vi "read header.vi"(6 "max bytes per line":i32=2048, 7 "max lines":i32=1024, 8 "error in (no error)":errorcluster, 11 "TCP Network Connection in":refnum<k5>) -> (0 "error out":errorcluster, 2 "header content":string, 3 "TCP Network Connection out":refnum<k5>)   [LabVIEW 2019, in "WebSocket Server Toolkit.lvlib"]
uses:
  WebSocket Server Toolkit.lvlib
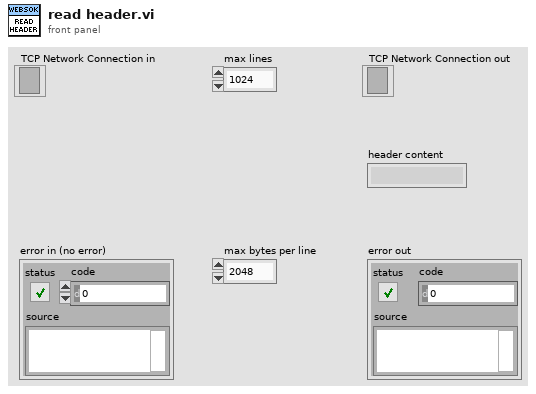
[diagram p1: front panel]
types:
  T1 = enum16{"Standard", "Buffered", "CRLF", "Immediate"}
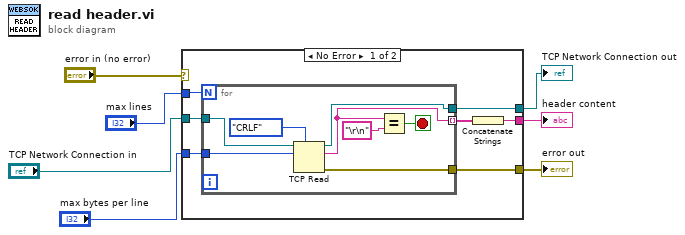
[diagram p0: block diagram]
diagram:
  n1 = case shown="No Error" "error in (no error)" {
    selector: "error in (no error)" -> [_ w23]
    tunnel: "TCP Network Connection in" -> [w14 w24]
    tunnel: [w12 _] -> w5
    tunnel: [w11 w23] -> w6
    tunnel: [w10 w24] -> w7
    tunnel: "max lines" -> [w9 _]
    tunnel: "max bytes per line" -> [w8 _]
    frame No Error {
      n2 = for {
        N: w9 -> [_]
        tunnel: w14 -> [w22]
        tunnel: [w20] -> w13 mode=indexing
        tunnel: [w18] -> w10
        tunnel: [w17] -> w11
        tunnel: w8 -> [w15]
        stop <- w16 stop-if-true
        n3 = TCP Read(connection ID=w22, bytes to read=w15, 7:T1."CRLF" ("mode (standard)")) -> (connection ID out=w18:refnum<k5>, data out=w20:string, error out=w17:errorcluster)  [unwired: 2 in]
        n4 = Equal?(x=w20, y="\r\n") -> (x = y?=w16:bool)
      }
      n5 = Concatenate Strings(w13) -> (w12:string)
    }
    frame Error {
    }
  }
  "TCP Network Connection out" <- w7
  "error out" <- w6
  "header content" <- w5
